vi "2_2_MNIST_Eval(FPGA)(PXI,sbRIO_Remote).vi"() -> ()   [LabVIEW 2020]
uses:
  <vilib>/userDefined/High Color/nirio_resource_hc.ctl
  Controls/Img_GrayScale.ctl
  <vilib>/FPGAPlugInAG/Dynamic/niLvFpga_Download_Dynamic.vi
  <vilib>/FPGAPlugInAG/Dynamic/niLvFpga_Run_Dynamic.vi
  <vilib>/Ngene/Deep Learning Toolkit/Toolkit/NN_Data/subVIs/Dataset/NN_Variant_to_DVR/4D/NN_Data_Variant_to_DVR(4D_SGL).vi
  <vilib>/Ngene/Deep Learning Toolkit/Toolkit/NN_Data/subVIs/Get_Data_Vals/4D/NN_Data_Get_ValByRef(4D_SGL_idx).vi
  <vilib>/Ngene/DeepLTK FPGA Addon/Toolkit/NNF_Host/API/NNF_Set_Input/NNF_Set_Input(3D_I8).vi
  <vilib>/Ngene/Deep Learning Toolkit/Toolkit/NN_Train/Eval_Loss/NN_Eval_Test_Error_Loss/NN_Eval(In3D_Out1D).vi
  <vilib>/Ngene/Deep Learning Toolkit/Toolkit/NN_Train/Eval_Loss/NN_Calc_Cofusion_Matrix/NN_Calc_Confusion_Matrix(In3D_Out1D).vi
  <vilib>/FPGAPlugInAG/Dynamic/niLvFpga_Close_Dynamic.vi
  <vilib>/rvi/interface/nirviMethod/nirviMethod.xnode
  <vilib>/rvi/interface/nirviCloseFPGA/nirviCloseFPGA.xnode
  <vilib>/Ngene/Deep Learning Toolkit/Toolkit/Deep_Learning_Toolkit_by_Ngene.lvlib
  <vilib>/Ngene/DeepLTK FPGA Addon/Toolkit/DeepLTK_FPGA_Addon.lvlib
  <vilib>/ptbypt/NI_PtbyPt.lvlib
panel:
  out "Incorrectly Classified Samples":T1[][](array[typedef])=[[{"image"=array28x28[784 elements], "Truth"=4, "Predicted"=9}, {"image"=array28x28[784 elements], "Truth"=2, "Predicted"=7}, {"image"=array28x28[784 elements], "Truth"=5, "Predicted"=3}, {"image"=array28x28[784 elements], "Truth"=9, "Predicted"=8}, {"image"=array28x28[784 elements], "Truth"=8, "Predicted"=9}, {"image"=array28x28[784 elements], "Truth"=8, "Predicted"=2}, {"image"=array28x28[784 elements], "Truth"=2, "Predicted"=1}, {"image"=array28x28[784 elements], "Truth"=5, "Predicted"=3}, {"image"=array28x28[784 elements], "Truth"=8, "Predicted"=9}, {"image"=array28x28[784 elements], "Truth"=6, "Predicted"=5}], [{"image"=array28x28[784 elements], "Truth"=7, "Predicted"=2}, {"image"=array28x28[784 elements], "Truth"=9, "Predicted"=4}, {"image"=array28x28[784 elements], "Truth"=9, "Predicted"=5}, {"image"=array28x28[784 elements], "Truth"=7, "Predicted"=1}, {"image"=array28x28[784 elements], "Truth"=5, "Predicted"=3}, {"image"=array28x28[784 elements], "Truth"=5, "Predicted"=3}, {"image"=array28x28[784 elements], "Truth"=9, "Predicted"=0}, {"image"=array28x28[784 elements], "Truth"=7, "Predicted"=1}, {"image"=array28x28[784 elements], "Truth"=9, "Predicted"=3}, {"image"=array28x28[784 elements], "Truth"=5, "Predicted"=3}], [{"image"=array28x28[784 elements], "Truth"=8, "Predicted"=3}, {"image"=array28x28[784 elements], "Truth"=9, "Predicted"=4}, {"image"=array28x28[784 elements], "Truth"=5, "Predicted"=3}, {"image"=array28x28[784 elements], "Truth"=7, "Predicted"=1}, {"image"=array28x28[784 elements], "Truth"=6, "Predicted"=0}, {"image"=array28x28[784 elements], "Truth"=9, "Predicted"=8}, {"image"=array28x28[784 elements], "Truth"=4, "Predicted"=9}, {"image"=array28x28[784 elements], "Truth"=9, "Predicted"=8}, {"image"=array28x28[784 elements], "Truth"=9, "Predicted"=4}, {"image"=array28x28[784 elements], "Truth"=2, "Predicted"=0}], [{"image"=array28x28[784 elements], "Truth"=2, "Predicted"=4}, {"image"=array28x28[784 elements], "Truth"=5, "Predicted"=3}, {"image"=array28x28[784 elements], "Truth"=6, "Predicted"=1}, {"image"=array28x28[784 elements], "Truth"=8, "Predicted"=0}, {"image"=array28x28[784 elements], "Truth"=3, "Predicted"=2}, {"image"=array28x28[784 elements], "Truth"=5, "Predicted"=3}, {"image"=array28x28[784 elements], "Truth"=6, "Predicted"=0}, {"image"=array28x28[784 elements], "Truth"=9, "Predicted"=4}, {"image"=array28x28[784 elements], "Truth"=7, "Predicted"=9}, {"image"=array28x28[784 elements], "Truth"=7, "Predicted"=2}], [{"image"=array28x28[784 elements], "Truth"=6, "Predicted"=0}, {"image"=array28x28[784 elements], "Truth"=9, "Predicted"=1}, {"image"=array28x28[784 elements], "Truth"=6, "Predicted"=4}, {"image"=array28x28[784 elements], "Truth"=5, "Predicted"=0}, {"image"=array28x28[784 elements], "Truth"=5, "Predicted"=3}, {"image"=array28x28[784 elements], "Truth"=7, "Predicted"=1}, {"image"=array28x28[784 elements], "Truth"=5, "Predicted"=3}, {"image"=array28x28[784 elements], "Truth"=9, "Predicted"=4}, {"image"=array28x28[784 elements], "Truth"=3, "Predicted"=2}, {"image"=array28x28[784 elements], "Truth"=2, "Predicted"=7}], [{"image"=array28x28[784 elements], "Truth"=6, "Predicted"=8}, {"image"=array28x28[784 elements], "Truth"=8, "Predicted"=3}, {"image"=array28x28[784 elements], "Truth"=5, "Predicted"=3}, {"image"=array28x28[784 elements], "Truth"=3, "Predicted"=8}, {"image"=array28x28[784 elements], "Truth"=9, "Predicted"=3}, {"image"=array28x28[784 elements], "Truth"=9, "Predicted"=8}, {"image"=array28x28[784 elements], "Truth"=9, "Predicted"=8}, {"image"=array28x28[784 elements], "Truth"=9, "Predicted"=7}, {"image"=array28x28[784 elements], "Truth"=7, "Predicted"=1}, {"image"=array28x28[784 elements], "Truth"=0, "Predicted"=7}], [{"image"=array28x28[784 elements], "Truth"=8, "Predicted"=1}, {"image"=array28x28[784 elements], "Truth"=2, "Predicted"=7}, {"image"=array28x28[784 elements], "Truth"=8, "Predicted"=6}, {"image"=array28x28[784 elements], "Truth"=7, "Predicted"=2}, {"image"=array28x28[784 elements], "Truth"=0, "Predicted"=1}, {"image"=array28x28[784 elements], "Truth"=2, "Predicted"=7}, {"image"=array28x28[784 elements], "Truth"=9, "Predicted"=4}, {"image"=array28x28[784 elements], "Truth"=5, "Predicted"=6}, {"image"=array28x28[784 elements], "Truth"=4, "Predicted"=9}, {"image"=array28x28[784 elements], "Truth"=5, "Predicted"=6}]]
  out "Dataset Size":i32=10000
  in  "FPGA Bitfile":path=path "D:/Ngene/GitHub/deepltk_fpga_examples/FPGA Bitfiles/NNF_sbRIO_9609_8Cores_120MHz.lvbitx"
  in  "FPGA Target":T2="rio://10.0.0.39/RIO0" caption="RIO Device"
  out "Speed (FPS)":dbl=63.28882399105552 format="%#_3p"
  out "Inference time(s)":dbl=0.015800578000016684 format="%#_3p"
  out "Iterations":i32=9999
  in  "Dataset":path
  out "Confusion Matrix":string[][](table)=[["978", "1", "0", "0", "0", "0", "0", "1", "0", "0", "0.9980"], ["0", "1135", "0", "0", "0", "0", "0", "0", "0", "0", "1.0000"], ["1", "1", "1025", "0", "1", "0", "0", "4", "0", "0", "0.9932"], ["0", "0", "2", "1007", "0", "0", "0", "0", "1", "0", "0.9970"], ["0", "0", "0", "0", "979", "0", "0", "0", "0", "3", "0.9969"], ["1", "0", "0", "11", "0", "878", "2", "0", "0", "0", "0.9843"], ["3", "1", "0", "0", "1", "1", "951", "0", "1", "0", "0.9927"], ["0", "5", "3", "0", "0", "0", "0", "1019", "0", "1", "0.9912"], ["1", "1", "1", "2", "0", "0", "1", "0", "966", "2", "0.9918"], ["1", "1", "0", "2", "6", "1", "0", "1", "5", "992", "0.9832"], ["0.9929", "0.9913", "0.9942", "0.9853", "0.9919", "0.9977", "0.9969", "0.9941", "0.9928", "0.9940", ""]]
  out "Error":sgl=0.007
  out "Loss":sgl=0.022489442
  in  "Weight File Path":path=path "D:/Ngene/GitHub/deepltk_fpga_examples/1_MNIST_Classification(PXI,sbRIO)/Models/1_Converted/mnist_cnn/NNF_mnist_cnn_weights_24_11_25__15_36_06.bin"
  in  "Configuration File Path":path=path "D:/Ngene/GitHub/deepltk_fpga_examples/1_MNIST_Classification(PXI,sbRIO)/Models/1_Converted/mnist_cnn/NNF_mnist_cnn_net_cfg_24_11_25__15_36_06.cfg"
  in  "Scalers File Path":path=path "D:/Ngene/GitHub/deepltk_fpga_examples/1_MNIST_Classification(PXI,sbRIO)/Models/1_Converted/mnist_cnn/NNF_mnist_cnn_net_scalers_24_11_25__15_36_06.cfg"
  # "Overview: This VI is designed to evaluate (measure the accuracy of) the model when executed on FPGA in PXI systems.\nThis VI can also be used to run the evaluation on sbRIO Targets remotely (from Windows based PC)\nRequirements: \n•DeepLTK - Deep Learning Toolkit for LabVIEW (https://www.ngene.co/deep-learning-toolkit-for-labview)\n•DeepLTK FPGA Addon (https://www.ngene.co/deepltk-accelerator-for-fpga)\nInstructions:\n1. Select FPGA target at FPGA Target control. PXI or remote sbRIO FPGA target can be specified.\n2. Provide path to compiled FPGA bitfile at FPGA Bitfile control.\n3. Provide the path to the dataset to be evaluated at Dataset. \n3. Provide paths to .cfg, .bin and scalers.cfg files generated during model conversion at Network Configuration File Path, Weight File Path and Scalers File Path controls.\n4. Run the VI with the default remaining settings.\n5. Observe measured accuracy at Loss, Error and Confusion Matrix indicators, and analyze Incorrectly Classified Samples.\n6. Press the Stop button to stop VI.\n7. To measure reference accuracy (when executed on CPU) run 2_1_MNIST_Eval(CPU,GPU).vi located in the project."
  # "Copy resource path from NI MAX if needed"
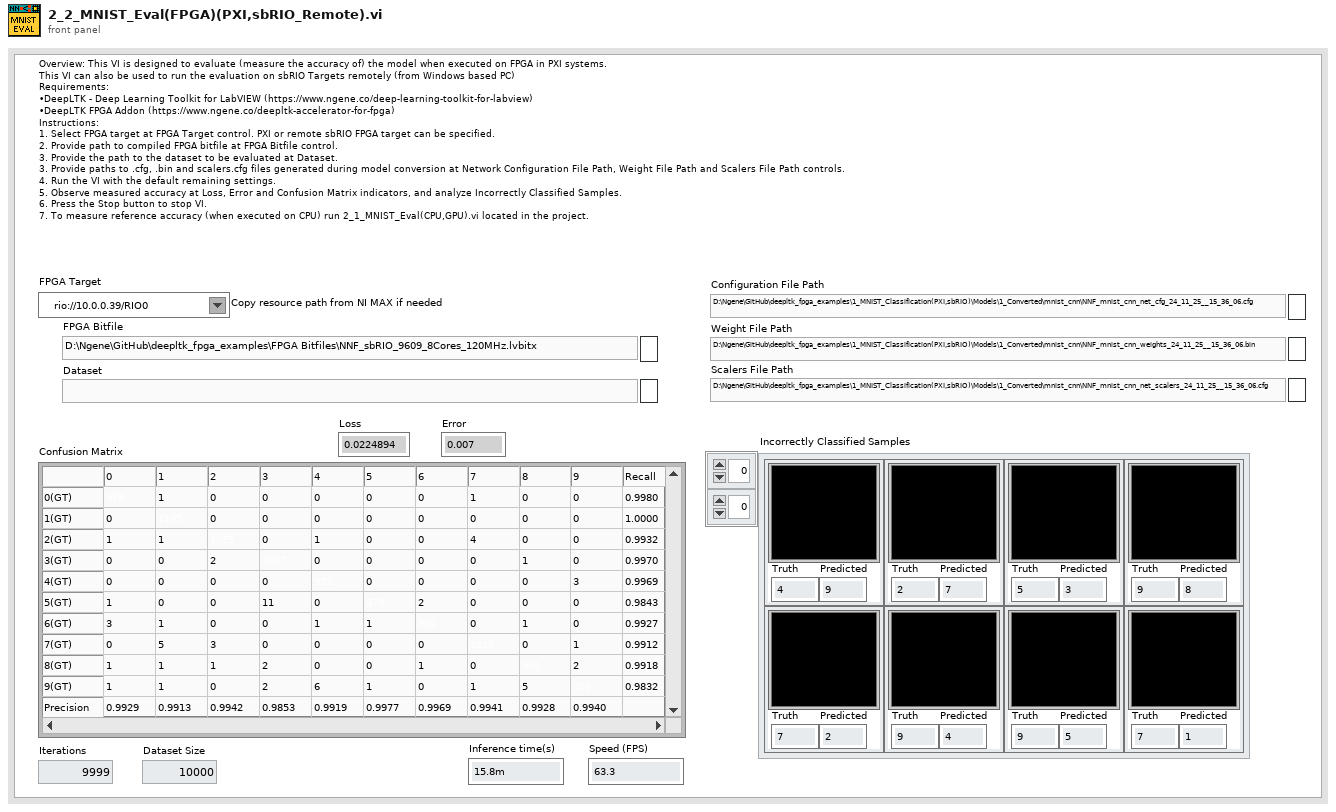
[diagram p1: front panel]
types:
  T1 = typedef "Img_GrayScale.ctl" = cluster{"image":sgl[][], "Truth":i32, "Predicted":i32}
  T2 = typedef "nirio_resource_hc.ctl" = tag
  T3 = typedef "Deep_Learning_Toolkit_by_Ngene.lvlib/NN_DataSets_All(In3D_Out1D).ctl" = cluster{"Train":T4, "Validation":T4, "Test":T4}
  T4 = typedef "Deep_Learning_Toolkit_by_Ngene.lvlib/NN_DataSet(In3D_Out1D).ctl" = cluster{"Inputs Ref.":variant, "Outputs Ref.":T5, "Dataset_Size":i32, "Dims_In":T6, "Dims_Out":i32, "Labels":string[], "File Paths":path[]}
  T5 = typedef "Deep_Learning_Toolkit_by_Ngene.lvlib/NN_Data_ref(2D_SGL).ctl" = refnum<data-value>
  T6 = typedef "Deep_Learning_Toolkit_by_Ngene.lvlib/NN_Dims(C,H,W).ctl" = cluster{"C":i32, "H":i32, "W":i32}
  T7 = typedef "DeepLTK_FPGA_Addon.lvlib/NNF.ctl" = cluster{"FPGA VI Ref ":refnum<k20>, "Subnets":T8[], "Dims_In":T6, "#Cores(enum)":T10, "NN_Ref":T11}
  T8 = typedef "DeepLTK_FPGA_Addon.lvlib/NNF_Subnet.ctl" = cluster{"Subnet Type":T9, "Subnet Data":variant, "Input Scaler":sgl, "Output Scaler":sgl}
  T9 = typedef "DeepLTK_FPGA_Addon.lvlib/NNF_Subnet_Type.ctl" = enum16{"CPU", "FPGA", "Split FPGA"}
  T10 = typedef "DeepLTK_FPGA_Addon.lvlib/NNF_No_Of_Cores.ctl" = enum16{"4CH", "8CH"}
  T11 = typedef "DeepLTK_FPGA_Addon.lvlib/NN_DVR.ctl" = refnum<data-value>
  T12 = typedef "Deep_Learning_Toolkit_by_Ngene.lvlib/NN_Data_ref(4D_SGL).ctl" = refnum<data-value>
  T13 = typedef "Deep_Learning_Toolkit_by_Ngene.lvlib/NN_Layer.ctl" = cluster{"Name":string, "Layer_Data":variant, "Layer_Type":T14, "Dims_In":T6, "Layers_In":variant, "Dims_Out":T6, "Layers_Out":variant, "Metrics":T15, "GPU_Data":variant, "mBatch":i32, "NN_Device":T16, "NNg_hdls":T17, "Train?":bool, "Dimty":T18, "RecptField":T19}
  T14 = typedef "Deep_Learning_Toolkit_by_Ngene.lvlib/NN_Layer_Type.ctl" = enum16{"Input1D", "Input3D", "Conv1D", "Conv2D", "Conv2D_Adv", "MaxPool", "AvgPool", "UpSample", "DropOut3D", "ShortCut", "Concat", "SoftMax3D", "FC", "DropOut", "Softmax", "Flatten", "YOLO_v2", "YOLO_v4", "Activation", "BatchNormalization", "Unsupported"}
  T15 = typedef "Deep_Learning_Toolkit_by_Ngene.lvlib/NN_Layer_Metrics.ctl" = cluster{"Data":dbl, "Params":dbl, "Ops":dbl}
  T16 = typedef "Deep_Learning_Toolkit_by_Ngene.lvlib/NN_Device.ctl" = enum16{"CPU", "GPU"}
  T17 = typedef "Deep_Learning_Toolkit_by_Ngene.lvlib/nng_cuda_handles.ctl" = cluster{"cudnn":u64, "cublas":u64, "stream":u64, "curand":u64}
  T18 = typedef "Deep_Learning_Toolkit_by_Ngene.lvlib/NN_Layer_Dimty.ctl" = enum16{"1D", "3D"}
  T19 = typedef "Deep_Learning_Toolkit_by_Ngene.lvlib/NN_Layer_RF_State.ctl" = cluster{"Dims":T20, "J":T20}
  T20 = typedef "Deep_Learning_Toolkit_by_Ngene.lvlib/NN_Dims(V,H).ctl" = cluster{"V":i32, "H":i32}
  T21 = typedef "Deep_Learning_Toolkit_by_Ngene.lvlib/NN.ctl" = cluster{"Name":string, "No of Layers":i32, "mBatch":i32, "Layers":T22[], "Dimty":T23, "Dims_In":T6, "Dims_Out":T6, "Working_Dir":path, "Train?":bool, "Train_Params":T24, "LR_Update_Policy":T27, "Session Data":T29, "Ground_truth":T30, "NNg_hdls":T17, "NN_Device":T16, "GPU Id":i32, "Labels":string[], "Receptive Field":T20[], "Loss_Type":T31, "Loss_Cfg_Prms":variant, "NNG_WS":T32}
  T22 = typedef "Deep_Learning_Toolkit_by_Ngene.lvlib/NN_Layer_ref.ctl" = refnum<data-value>
  T23 = typedef "Deep_Learning_Toolkit_by_Ngene.lvlib/NN_In_Out_Dim-ty.ctl" = enum8{"In1D_Out1D", "In3D_Out1D", "In3D_Out3D", "In3D_OutBBox"}
  T24 = typedef "Deep_Learning_Toolkit_by_Ngene.lvlib/NN_Train_Params.ctl" = cluster{"Optimizer":T25, "Beta_1":sgl, "Beta_2":sgl, "Weight Decay(L1)":sgl, "Weight Decay(L2)":sgl, "Data_Sampling":T26}
  T25 = typedef "Deep_Learning_Toolkit_by_Ngene.lvlib/NN_Train_Optimizer.ctl" = enum16{"SGD", "Adam", "Adagrad", "Adadelta", "RMSProp", "Nesterov"}
  T26 = typedef "Deep_Learning_Toolkit_by_Ngene.lvlib/NN_Train_Data_Sampling.ctl" = enum16{"Random", "Sequential"}
  T27 = typedef "Deep_Learning_Toolkit_by_Ngene.lvlib/NN_LR_Policy_Cfg.ctl" = cluster{"Policy_Type":T28, "LR0":dbl, "k":sgl, "WarmUp_Policy":enum16{"Step", "Ramp"}, "WarmUp_Iter":i32, "WarmUp_Ratio":sgl}
  T28 = typedef "Deep_Learning_Toolkit_by_Ngene.lvlib/NN_LR_Policy_Type.ctl" = enum16{"Manual", "Step", "Exp", "1/t"}
  T29 = typedef "Deep_Learning_Toolkit_by_Ngene.lvlib/NN_Train_Session_Data.ctl" = cluster{"Epochs":sgl, "Tot_Iter":i32, "LR":sgl, "LR_iter":i32}
  T30 = typedef "Deep_Learning_Toolkit_by_Ngene.lvlib/NN_Ground_truth.ctl" = cluster{"Y":variant}
  T31 = typedef "Deep_Learning_Toolkit_by_Ngene.lvlib/NN_Loss_Type.ctl" = enum16{"None", "MSE", "CrossEntropy", "YOLO_v2", "YOLO_v4"}
  T32 = typedef "Deep_Learning_Toolkit_by_Ngene.lvlib/NNG_WS.ctl" = cluster{"NNG_WS_Mem":T33, "Max_WS_Size":i64}
  T33 = typedef "Deep_Learning_Toolkit_by_Ngene.lvlib/NNg_WS_Mem_DVR.ctl" = refnum<data-value>
  T34 = typedef "Deep_Learning_Toolkit_by_Ngene.lvlib/NN_Eval_Params.ctl" = cluster{"Loss":sgl, "Error":sgl}
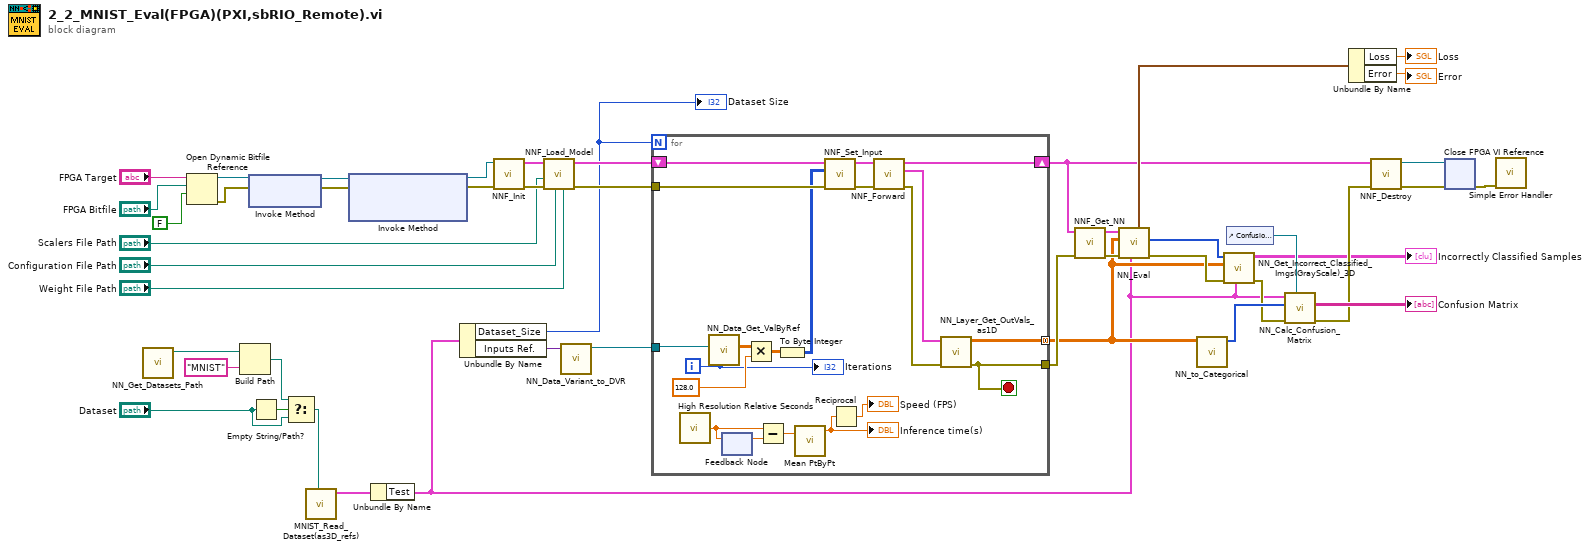
[diagram p0: block diagram]
diagram:
  n1 = call "NN_Get_Datasets_Path.vi"() -> ("Datasets path"=w3:path)  [unwired: 11 in]
  n2 = Open Dynamic Bitfile Reference(0:"FPGA Target", 1:"FPGA Bitfile", 2:FALSE ("Run When Loaded")) -> (5:w24:refnum<k20>, 8:w22:errorcluster)  [unwired: 2 in]
  n3 = Build Path(base path=w3, name or relative path="MNIST") -> (appended path=w5:path)
  n4 = xnode "Invoke Method"("FPGA VI Reference In"=w24, "error in"=w22) -> ("FPGA VI Reference Out"=w23:refnum<k20>, "error out"=w21:errorcluster)
  n5 = Empty String/Path?(string/path="Dataset") -> (empty?=w4:bool)
  n6 = Select(t=w5, s=w4, f="Dataset") -> (s? t:f=w1:path)
  n7 = call "MNIST_Read_Dataset(as3D_refs).vi"("MNIST Dataset Path"=w1) -> ("Data(3D)_Refs"=w26:T3)  [unwired: 9 in, 1 out]
  n8 = xnode "Invoke Method"("FPGA VI Reference In"=w23, "error in"=w21) -> ("FPGA VI Reference Out"=w27:refnum<k20>, "error out"=w42:errorcluster)  [unwired: 1 in]
  n9 = Unbundle By Name(w26) -> ("Test"=w9:T4)
  n10 = Unbundle By Name(w9) -> ("Dataset_Size"=w18:i32, "Inputs Ref."=w37:variant)
  "Dataset Size" <- w18
  n11 = call <vilib>:"NNF_Init.vi"("error in"=w42, "FPGA Interface"=w27) -> ("error out"=w45:errorcluster, "NNF out"=w44:T7)  [unwired: 7 in, 1 out]
  n12 = call <vilib>:"NNF_Load_Model.vi"("Weight File Path"="Weight File Path", "Network CFG File Path"="Configuration File Path", "Error in"=w45, "Scalers"="Scalers File Path", "NNF in"=w44) -> ("error Out"=w35:errorcluster, "NNF out"=w33:T7)  [unwired: 5 in]
  n13 = call-poly <vilib>:"NN_Data_Variant_to_DVR.vi"("Inputs Ref."=w37) -> ("DVR(4D_SGL)"=w29:T12)  [unwired: 9 in, 1 out]
  n14 = for {
    N: w18 -> [_]
    shift-right: [w65] -> w8
    shift-left: w33 -> [w64]
    tunnel: w29 -> [w63]
    tunnel: [w53] -> w12 mode=concatenating
    tunnel: [w54] -> w36
    tunnel: w35 -> [w57]
    i -> [w51]
    stop <- w54 stop-if-true
    n15 = call <vilib>:"High Resolution Relative Seconds.vi"() -> ("relative seconds"=w46:dbl)
    n16 = call-poly <vilib>:"NN_Data_Get_ValByRef.vi"("index (vol)"=w51, "DVR(4D_SGL)"=w63) -> ("Value(3D_SGL)"=w62:sgl[][][])  [unwired: 6 in, 1 out]
    n17 = feedback #1() -> (w47:dbl)  [unwired: 1 in]
    n18 = feedback-in #1(w46) -> ()
    n19 = Multiply(x=w62, y=sgl 128.0 ("x")) -> (x*y=w58:sgl[][][])
    n20 = Subtract(x=w46, y=w47) -> (x-y=w49:dbl)
    n21 = To Byte Integer(number=w58) -> (8bit integer=w52:i8[][][])
    n22 = call <vilib>:"Mean PtByPt.vi"("x"=w49) -> ("mean"=w48:dbl)  [unwired: 3 in, 1 out]
    "Inference time(s)" <- w48
    n23 = call-poly <vilib>:"NNF_Set_Input.vi"("error in"=w57, "Data_in(3D_I8)"=w52, "NNF in"=w64) -> ("error out"=w59:errorcluster, "NNF out"=w60:T7)  [unwired: 7 in]
    n24 = Reciprocal(x=w48) -> (1/x=→"Speed (FPS)":dbl)
    n25 = call <vilib>:"NNF_Forward.vi"("error in"=w59, "NNF in"=w60) -> ("error out"=w55:errorcluster, "Last_Layer"=w56:T13, "NNF out"=w65:T7)  [unwired: 7 in]
    n26 = call <vilib>:"NN_Layer_Get_OutVals_as1D.vi"("error in (no error)"=w55, "Layer"=w56) -> ("error out"=w54:errorcluster, "Out(as1D)"=w53:sgl[][])  [unwired: 8 in]
    "Iterations" <- w51
  }
  n27 = call "NNF_Get_NN.vi"("NNF in"=w8) -> ("NN out"=w7:T21)  [unwired: 10 in]
  n28 = call-poly <vilib>:"NN_Eval.vi"("Dataset"=w9, "error in (no error)"=w36, "Predictions"=w12, "NN in"=w7) -> ("error out"=w14:errorcluster, "Incrct_Class_idx"=w15:i32[], "NN_Eval_Params"=w32:T34)  [unwired: 4 in, 1 out]
  n29 = call <vilib>:"NN_to_Categorical.vi"("Prediction"=w12) -> ("Label_Idx"=w28:i32[])  [unwired: 10 in]
  n30 = call "NN_Get_Incorrect_Classified_Imgs(GrayScale)_3D.vi"("Test_Data"=w9, "error in (no error)"=w14, "Predictions"=w12, "MisClassed_idx"=w15) -> ("error out"=w13:errorcluster, "Images(GrayScale)"=→"Incorrectly Classified Samples":T1[][])  [unwired: 6 in]
  n31 = control-ref of="Confusion Matrix"() -> (w19:refnum<vi>)
  n32 = call-poly <vilib>:"NN_Calc_Confusion_Matrix.vi"("Confusion Matrix (Table) ref."=w19, "error in (no error)"=w13, "Predictions"=w28, "Dataset"=w9) -> ("error out"=w11:errorcluster, "Confusion Matrix (Table)"=→"Confusion Matrix":string[][])  [unwired: 3 in, 3 out]
  n33 = Unbundle By Name(w32) -> ("Loss"=→"Loss":sgl, "Error"=→"Error":sgl)
  n34 = call <vilib>:"NNF_Destroy.vi"("error in"=w11, "NNF in"=w8) -> ("error out"=w41:errorcluster, "FPGA VI Ref"=w40:refnum<k20>)  [unwired: 8 in]
  n35 = xnode "Close FPGA VI Reference"("FPGA VI Reference In"=w40, "error in"=w41) -> ("error out"=w39:errorcluster)
  n36 = call <vilib>:"Simple Error Handler.vi"("error in (no error)"=w39) -> ()  [unwired: 4 in, 5 out]
